vi "Call_EXE.vi"() -> ()   [LabVIEW 2014]
panel:
  out "standard error":string
  in  "command line":string="/home/pi/hello"
  out "standard output":string
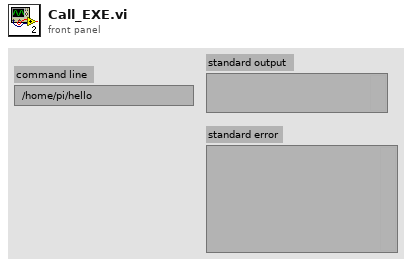
[diagram p1: front panel]
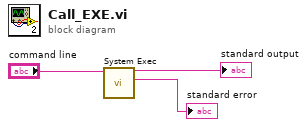
[diagram p0: block diagram]
diagram:
  n1 = call <vilib>:"System Exec.vi"("command line"="command line") -> ("standard error"=→"standard error":string, "standard output"=→"standard output":string)  [unwired: 7 in, 2 out]
